vi "dfd_Convert All Quantizers to String.vi"(5 "indent order":i32, 7 "filter type":T1, 10 "Gain on Target?":bool, 11 "quantization settings":T2[](array[typedef]) {"source" items=["Coef a/k"=0, "Coef b/v"=7, "Input"=1, "Output"=2, "Multiplicand"=3, "Product"=4, "Sum"=5, "Delay"=6, "Gain"=8]}) -> (3 "string out":string)   [LabVIEW 2017, in "NI_DigFilter_Process.lvlib"]
uses:
  <vilib>/addons/Digital Filter Design/NI_DigFilter_Process.lvlib
  <vilib>/addons/Digital Filter Design/_Objects.llb/dfd_Internal Quantization Settings.ctl
  <vilib>/addons/Digital Filter Design/_Objects.llb/dfd_Internal Quantization Srcs.ctl
  <vilib>/addons/Digital Filter Design/_Objects.llb/DFD Filter Structure Type Selector.ctl
  <vilib>/addons/Digital Filter Design/NI_DigFilterLicensed.lvlib
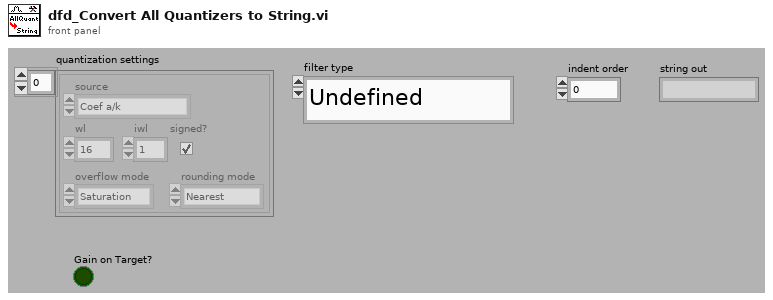
[diagram p1: front panel]
types:
  T1 = typedef "NI_DigFilterLicensed.lvlib/DFD Filter Structure Type Selector.ctl" = enum16{"Undefined", "FIR Direct Form", "FIR Direct Form Transposed", "FIR Symmetric", "FIR Antisymmetric", "IIR Direct Form I", "IIR Direct Form I Transposed", "IIR Direct Form II", "IIR Direct Form II Transposed", "IIR Cascaded Second Order Sections Form I", "IIR Cascaded Second Order Sections Form I Transposed", "IIR Cascaded Second Order Sections Form II", "IIR Cascaded Second Order Sections Form II Transposed", "Lattice Allpass (basic sections)", "Lattice Allpass (one multiplier sections)", "Lattice Allpass (normalized sections)", "Lattice AR (basic sections)", "Lattice AR (one multiplier sections)", "Lattice AR (normalized sections)", "Lattice MA (minimum phase)", "Lattice MA (maximum phase)", "Lattice ARMA (basic sections)", "Lattice ARMA (one multiplier sections)", "Lattice ARMA (normalized sections)"}
  T2 = typedef "NI_DigFilterLicensed.lvlib/dfd_Internal Quantization Settings.ctl" = cluster{"source":T3, "wl":i16, "iwl":i16, "overflow mode":enum16{"Saturation", "Wrap"}, "rounding mode":enum16{"Nearest", "Truncation"}, "signed?":bool}
  T3 = typedef "NI_DigFilterLicensed.lvlib/dfd_Internal Quantization Srcs.ctl" = u16
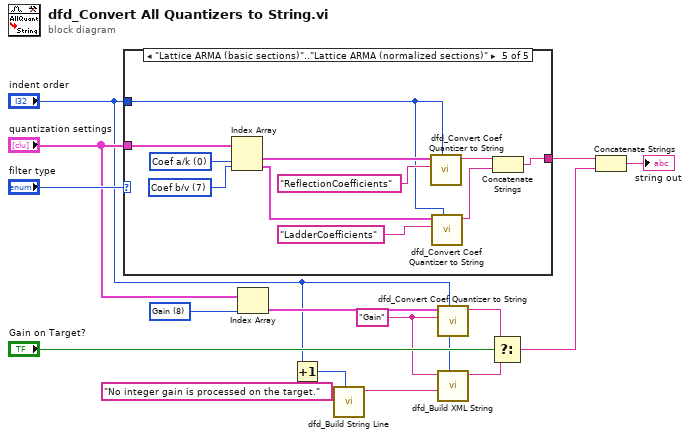
[diagram p0: block diagram]
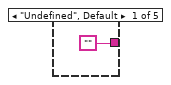
[diagram p2: hidden frame]
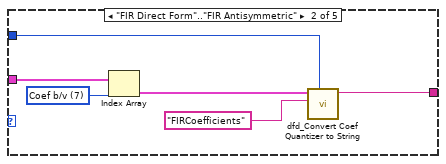
[diagram p3: hidden frame]
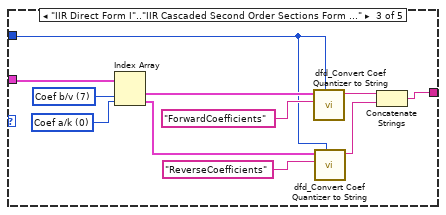
[diagram p4: hidden frame]
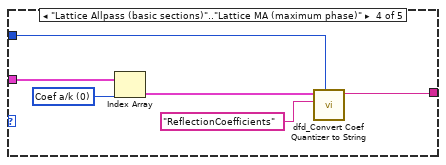
[diagram p5: hidden frame]
diagram:
  w7 = "Gain"
  w14 = T3 8 items=["Coef a/k"=0, "Coef b/v"=7, "Input"=1, "Output"=2, "Multiplicand"=3, "Product"=4, "Sum"=5, "Delay"=6, "Gain"=8] ("source")
  n1 = case shown="\"Lattice ARMA (basic sections)\"..\"Lattice ARMA (normalized sections)\"" "filter type" {
    tunnel: "quantization settings" -> [_ w21 w30 w35 w43]
    tunnel: "indent order" -> [_ w22 w26 w36 w44]
    tunnel: ["" w17 w25 w34 w40] -> w12
    frame "Undefined", Default {
    }
    frame "FIR Direct Form".."FIR Antisymmetric" {
      w20 = T3 7 items=["Coef a/k"=0, "Coef b/v"=7, "Input"=1, "Output"=2, "Multiplicand"=3, "Product"=4, "Sum"=5, "Delay"=6, "Gain"=8] ("source")
      n2 = Index Array(array=w21, index=w20) -> (element=w19:T2)
      n3 = call <vilib>:"dfd_Convert Coef Quantizer to String.vi"("indent order"=w22, "quantizer name"="FIRCoefficients", "quantization settings"=w19) -> ("xml string out"=w17:string)  [unwired: 8 out]
    }
    frame "IIR Direct Form I".."IIR Cascaded Second Order Sections Form II Transposed" {
      w29 = T3 0 items=["Coef a/k"=0, "Coef b/v"=7, "Input"=1, "Output"=2, "Multiplicand"=3, "Product"=4, "Sum"=5, "Delay"=6, "Gain"=8] ("source")
      w33 = T3 7 items=["Coef a/k"=0, "Coef b/v"=7, "Input"=1, "Output"=2, "Multiplicand"=3, "Product"=4, "Sum"=5, "Delay"=6, "Gain"=8] ("source")
      n4 = Index Array(array=w30, index #1=w33, index #2=w29) -> (element #1=w32:T2, element #2=w28:T2)
      n5 = call <vilib>:"dfd_Convert Coef Quantizer to String.vi"("indent order"=w26, "quantizer name"="ForwardCoefficients", "quantization settings"=w32) -> ("xml string out"=w24:string)  [unwired: 8 out]
      n6 = call <vilib>:"dfd_Convert Coef Quantizer to String.vi"("indent order"=w26, "quantizer name"="ReverseCoefficients", "quantization settings"=w28) -> ("xml string out"=w23:string)  [unwired: 8 out]
      n7 = Concatenate Strings(w24, w23) -> (w25:string)
    }
    frame "Lattice Allpass (basic sections)".."Lattice MA (maximum phase)" {
      w39 = T3 0 items=["Coef a/k"=0, "Coef b/v"=7, "Input"=1, "Output"=2, "Multiplicand"=3, "Product"=4, "Sum"=5, "Delay"=6, "Gain"=8] ("source")
      n8 = Index Array(array=w35, index=w39) -> (element=w38:T2)
      n9 = call <vilib>:"dfd_Convert Coef Quantizer to String.vi"("indent order"=w36, "quantizer name"="ReflectionCoefficients", "quantization settings"=w38) -> ("xml string out"=w34:string)  [unwired: 8 out]
    }
    frame "Lattice ARMA (basic sections)".."Lattice ARMA (normalized sections)" {
      w47 = T3 7 items=["Coef a/k"=0, "Coef b/v"=7, "Input"=1, "Output"=2, "Multiplicand"=3, "Product"=4, "Sum"=5, "Delay"=6, "Gain"=8] ("source")
      w50 = T3 0 items=["Coef a/k"=0, "Coef b/v"=7, "Input"=1, "Output"=2, "Multiplicand"=3, "Product"=4, "Sum"=5, "Delay"=6, "Gain"=8] ("source")
      n10 = Index Array(array=w43, index #1=w50, index #2=w47) -> (element #1=w49:T2, element #2=w46:T2)
      n11 = call <vilib>:"dfd_Convert Coef Quantizer to String.vi"("indent order"=w44, "quantizer name"="ReflectionCoefficients", "quantization settings"=w49) -> ("xml string out"=w42:string)  [unwired: 8 out]
      n12 = call <vilib>:"dfd_Convert Coef Quantizer to String.vi"("indent order"=w44, "quantizer name"="LadderCoefficients", "quantization settings"=w46) -> ("xml string out"=w41:string)  [unwired: 8 out]
      n13 = Concatenate Strings(w42, w41) -> (w40:string)
    }
  }
  n14 = Index Array(array="quantization settings", index=w14) -> (element=w13:T2)
  n15 = Increment(x="indent order") -> (x+1=w5:i32)
  n16 = call <vilib>:"dfd_Build String Line.vi"("indent order"=w5, "string"="No integer gain is processed on the target.") -> ("string line"=w4:string)  [unwired: 9 out]
  n17 = call <vilib>:"dfd_Convert Coef Quantizer to String.vi"("indent order"="indent order", "quantizer name"=w7, "quantization settings"=w13) -> ("xml string out"=w9:string)  [unwired: 8 out]
  n18 = call <vilib>:"dfd_Build XML String.vi"("indent order"="indent order", "string in"=w4, "element name"=w7) -> ("xml string out"=w6:string)  [unwired: 1 in, 7 out]
  n19 = Select(t=w9, s="Gain on Target?", f=w6) -> (s? t:f=w8:string)
  n20 = Concatenate Strings(w12, w8) -> (→"string out":string)
